vi "CreateDiagram.vi"(6 "UID":i32, 7 "PythonConverter in":refnum<class "PythonBDConverter.lvclass">, 8 "error in":errorcluster, 11 "VI Interpreter in":refnum<class "VI Interpreter.lvclass">) -> (0 "error out":errorcluster, 3 "VI Interpreter out":refnum<class "VI Interpreter.lvclass">, 5 "PythonConverter out":refnum<class "PythonBDConverter.lvclass">)   [LabVIEW 2014, in "PythonBDConverter.lvclass"]
uses:
  PythonBDConverter.lvclass
  VI Interpreter/Classes/VI Interpreter/VI Interpreter.lvclass
  VI Interpreter/Classes/Diagram/Diagram.lvclass
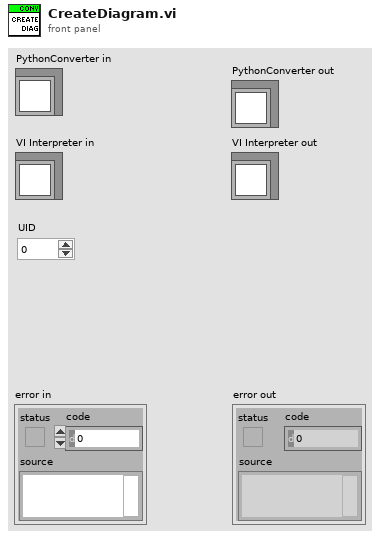
[diagram p1: front panel]
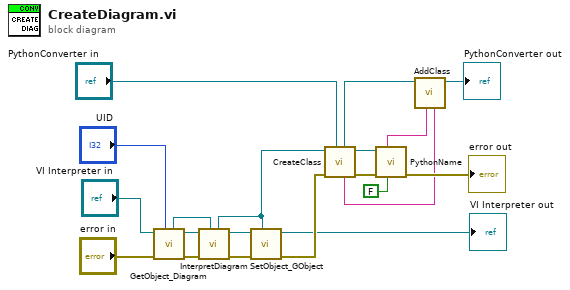
[diagram p0: block diagram]
diagram:
  n1 = call "GetObject_Diagram.vi"("UID"="UID", "error in"="error in", "VI Interpreter in"="VI Interpreter in") -> ("error out"=w5:errorcluster, "VI Interpreter out"=w6:refnum<class "VI Interpreter.lvclass">, "Diagram"=w4:refnum<class "Diagram.lvclass">)  [unwired: 3 in, 1 out]
  n2 = call "InterpretDiagram.vi"("Diagram"=w4, "error in"=w5, "VI Interpreter in"=w6) -> ("error out"=w8:errorcluster, "VI Interpreter out"=w7:refnum<class "VI Interpreter.lvclass">, "Diagram out"=w3:refnum<class "Diagram.lvclass">)  [unwired: 4 in]
  n3 = call "SetObject_GObject.vi"("GObject"=w3, "error in"=w8, "VI Interpreter in"=w7) -> ("error out"=w2:errorcluster, "VI Interpreter out"=→"VI Interpreter out":refnum<class "VI Interpreter.lvclass">)  [unwired: 5 in]
  n4 = call-dynamic "CreateClass.vi"("PythonConverter in"="PythonConverter in", "error in"=w2, "Diagram in"=w3) -> ("error out"=w15:errorcluster, "Diagram out"=w16:refnum<class "Diagram.lvclass">, "diagram"=w9:string, "PythonConverter out"=w17:refnum<class "PythonBDConverter.lvclass">)  [unwired: 5 in]
  n5 = call-dynamic "PythonName.vi"("add self"=FALSE, "error in"=w15, "Diagram in"=w16) -> ("error out"=→"error out":errorcluster, "UID"=w14:string)  [unwired: 5 in, 2 out]
  n6 = call "AddClass.vi"("definition"=w9, "name"=w14, "PythonConverter in"=w17) -> ("PythonConverter out"=→"PythonConverter out":refnum<class "PythonBDConverter.lvclass">)  [unwired: 5 in, 1 out]
